vi "Create BooleanMessage.vi"(8 "error in (no error)":errorcluster, 10 "Message Data":bool, 11 "Message Name":string) -> (0 "error out":errorcluster, 3 "BooleanMessage out":refnum<class "BooleanMessage.lvclass">)   [LabVIEW 2009, in "LapDog.Messaging.v2.NativeTypes.lvlib" / "BooleanMessage.lvclass"]
doc: "Returns a BooleanMessage object with the given name.\n\nThis method executes regardless of the error in state."
uses:
  BooleanMessage.lvclass
  BooleanMessage.lvclass/BooleanMessage.ctl
  Messaging.v2/MessageObject/Message.lvclass
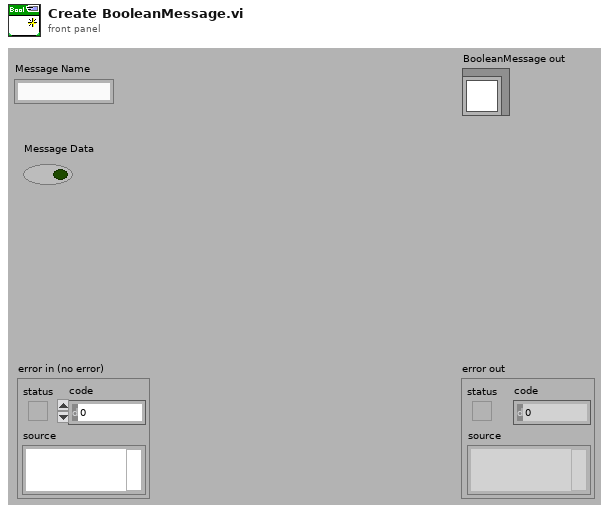
[diagram p1: front panel]
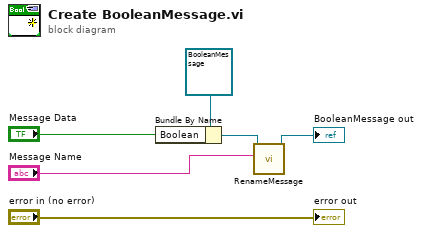
[diagram p0: block diagram]
diagram:
  n1 = Bundle By Name(cluster=refnum<class "BooleanMessage.lvclass"> refnum ("BooleanMessage in"), "Boolean"="Message Data") -> (w3:refnum<class "BooleanMessage.lvclass">)
  n2 = call "RenameMessage.vi"("Message Name"="Message Name", "Message in"=w3) -> ("Message out"=→"BooleanMessage out":refnum<class "BooleanMessage.lvclass">)  [unwired: 8 in, 1 out]
  "error out" <- "error in (no error)"
